vi "DCA Convert Range and Resolution.vi"(2 "Resolution":T3, 3 "Range":T4) -> (0 "Converted Resolution":T1, 1 "Converted Range":T2)   [LabVIEW 2011]
uses:
  TypeDefs/DCA Range.ctl
  TypeDefs/DCA Resolution.ctl
  drivers/DMM/Agilent/TypeDefs/Agilent DMM Range.ctl
  drivers/DMM/Agilent/TypeDefs/Agilent DMM Resolution.ctl
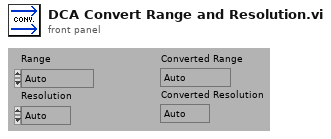
[diagram p1: front panel]
types:
  T1 = typedef "Agilent DMM Resolution.ctl" = enum16{"Auto", "Min", "Max", "4 1/2", "5 1/2", "6 1/2"}
  T2 = typedef "Agilent DMM Range.ctl" = enum16{"Auto", "Min", "Max", "0.01", "0.1", "1", "3", "10", "100", "1,000", "10,000", "100,000", "1,000,000", "10,000,000", "100,000,000"}
  T3 = typedef "DCA Resolution.ctl" = enum16{"Auto", "4 1/2", "5 1/2", "6 1/2"}
  T4 = typedef "DCA Range.ctl" = enum16{"Auto", "Minimum", "Maximum", "100", "1,000", "10,000", "100,000", "1,000,000", "10,000,000", "100,000,000"}
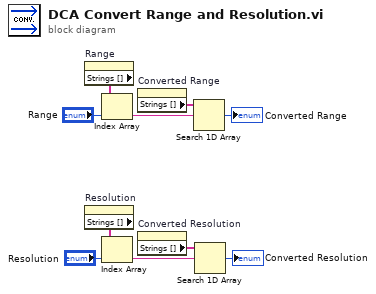
[diagram p0: block diagram]
diagram:
  n1 = property on="Range" class="Enum (strict)"() -> ("Strings []"=w9:string[])  [unwired: 2 in, 2 out]
  n2 = property on="Resolution" class="Enum (strict)"() -> ("Strings []"=w4:string[])  [unwired: 2 in, 2 out]
  n3 = Index Array(array=w9, index="Range") -> (element=w7:string)
  n4 = Index Array(array=w4, index="Resolution") -> (element=w2:string)
  n5 = property on="Converted Range" class="Enum (strict)"() -> ("Strings []"=w10:string[])  [unwired: 2 in, 2 out]
  n6 = property on="Converted Resolution" class="Enum (strict)"() -> ("Strings []"=w3:string[])  [unwired: 2 in, 2 out]
  n7 = Search 1D Array(1D array=w10, element=w7) -> (index of element=→"Converted Range":i32)  [unwired: 1 in]
  n8 = Search 1D Array(1D array=w3, element=w2) -> (index of element=→"Converted Resolution":i32)  [unwired: 1 in]
